vi "Path Crossing XY Plane.vi"(8 "error in (no error)":errorcluster, 9 "Limits":cluster{"Min":ext, "Max":ext}, 10 "Hailstone 2":refnum<class "Hailstone.lvclass">, 11 "Hailstone In":refnum<class "Hailstone.lvclass">) -> (0 "error out":errorcluster, 2 "Crossing?":bool, 3 "Hailstone Out":refnum<class "Hailstone.lvclass">)   [LabVIEW 2021, in "Hailstone.lvclass"]
uses:
  Hailstone.lvclass
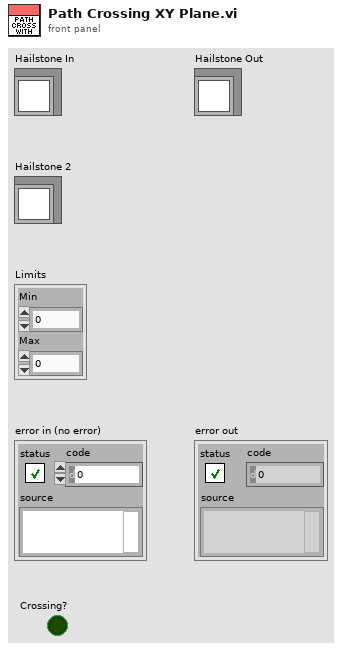
[diagram p1: front panel]
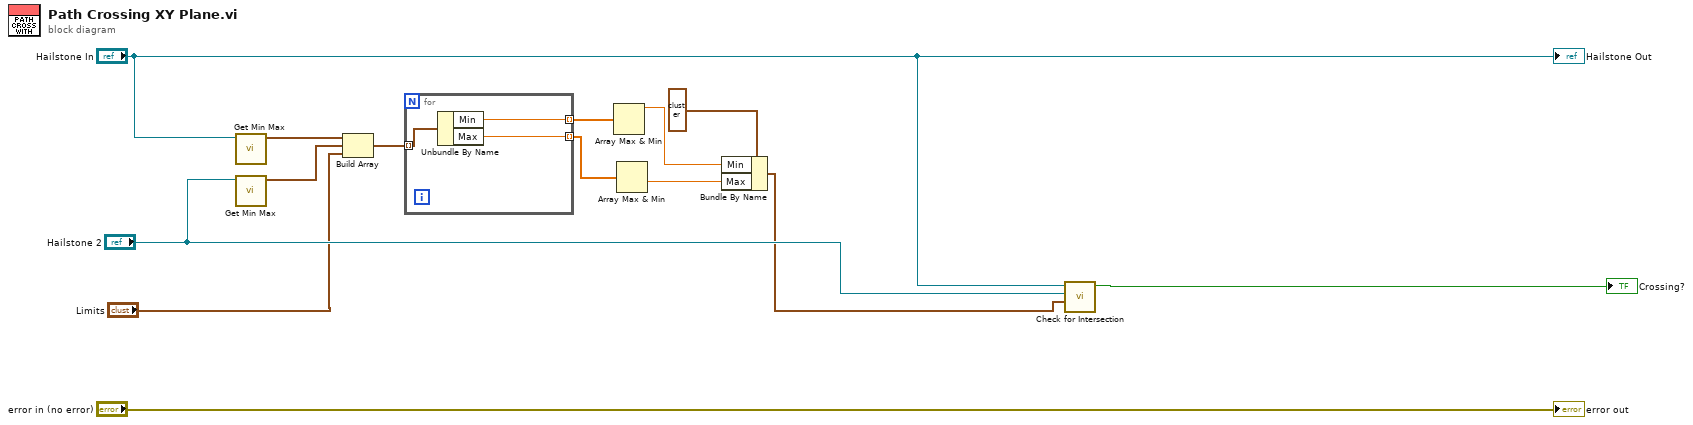
[diagram p0: block diagram]
diagram:
  n1 = call "Get Min Max.vi"("Hailstone in"="Hailstone In") -> ("Limits"=w10:cluster{"Min":ext, "Max":ext})  [unwired: 10 in]
  n2 = call "Get Min Max.vi"("Hailstone in"="Hailstone 2") -> ("Limits"=w9:cluster{"Min":ext, "Max":ext})  [unwired: 10 in]
  n3 = Build Array(w10, w9, "Limits") -> (w8:cluster{"Min":ext, "Max":ext}[])
  n4 = for {
    tunnel: w8 -> [w17] mode=indexing
    tunnel: [w16] -> w7 mode=indexing
    tunnel: [w15] -> w6 mode=indexing
    n5 = Unbundle By Name(w17) -> ("Min"=w16:ext, "Max"=w15:ext)
  }
  n6 = Array Max & Min(array=w7) -> (max value=w4:ext)  [unwired: 3 out]
  n7 = Array Max & Min(array=w6) -> (min value=w3:ext)  [unwired: 3 out]
  n8 = Bundle By Name(cluster=cluster{"Min":ext, "Max":ext} {"Min"=0.0, "Max"=0.0} ("Limits"), "Min"=w4, "Max"=w3) -> (w1:cluster{"Min":ext, "Max":ext})
  n9 = call "Check for Intersection.vi"("Limits in"=w1, "Hailstone 2"="Hailstone 2", "Hailstone in"="Hailstone In") -> ("Boolean"=→"Crossing?":bool)  [unwired: 8 in]
  "error out" <- "error in (no error)"
  "Hailstone Out" <- "Hailstone In"
